vi "Utilization.vi"() -> ()   [LabVIEW 2012]
uses:
  <vilib>/addons/database/Auxilliary.llb/DB Tools Cursor Type.ctl
  <vilib>/addons/database/Connection.llb/DB Tools Open Connec (Path).vi
  <vilib>/addons/database/Connection.llb/Conn Execute.vi
  <vilib>/addons/database/Recordset.llb/Rec Fetch Recordset Data (R).vi
  <vilib>/addons/database/Recordset.llb/Rec Destroy - Connection.vi
  <vilib>/addons/database/_DB Variant To Data/Database Variant To Data.xnode
  <vilib>/addons/database/NI_Database_API.lvlib
panel:
  out "sum":dbl
  out "array":dbl[](array[numeric])
  out "data 6":string
  out "Minutes 3":i32
  out "Minutes 2":i32
  out "Numeric 2":i32
  out "Numeric":i32
  out "Minutes":i32
  out "data 5":string
  out "data 4":string
  out "data 3":string
  out "data 2":string
  out "data":string
  out "recordset data":variant[][](array[variant])
  out "error out":errorcluster
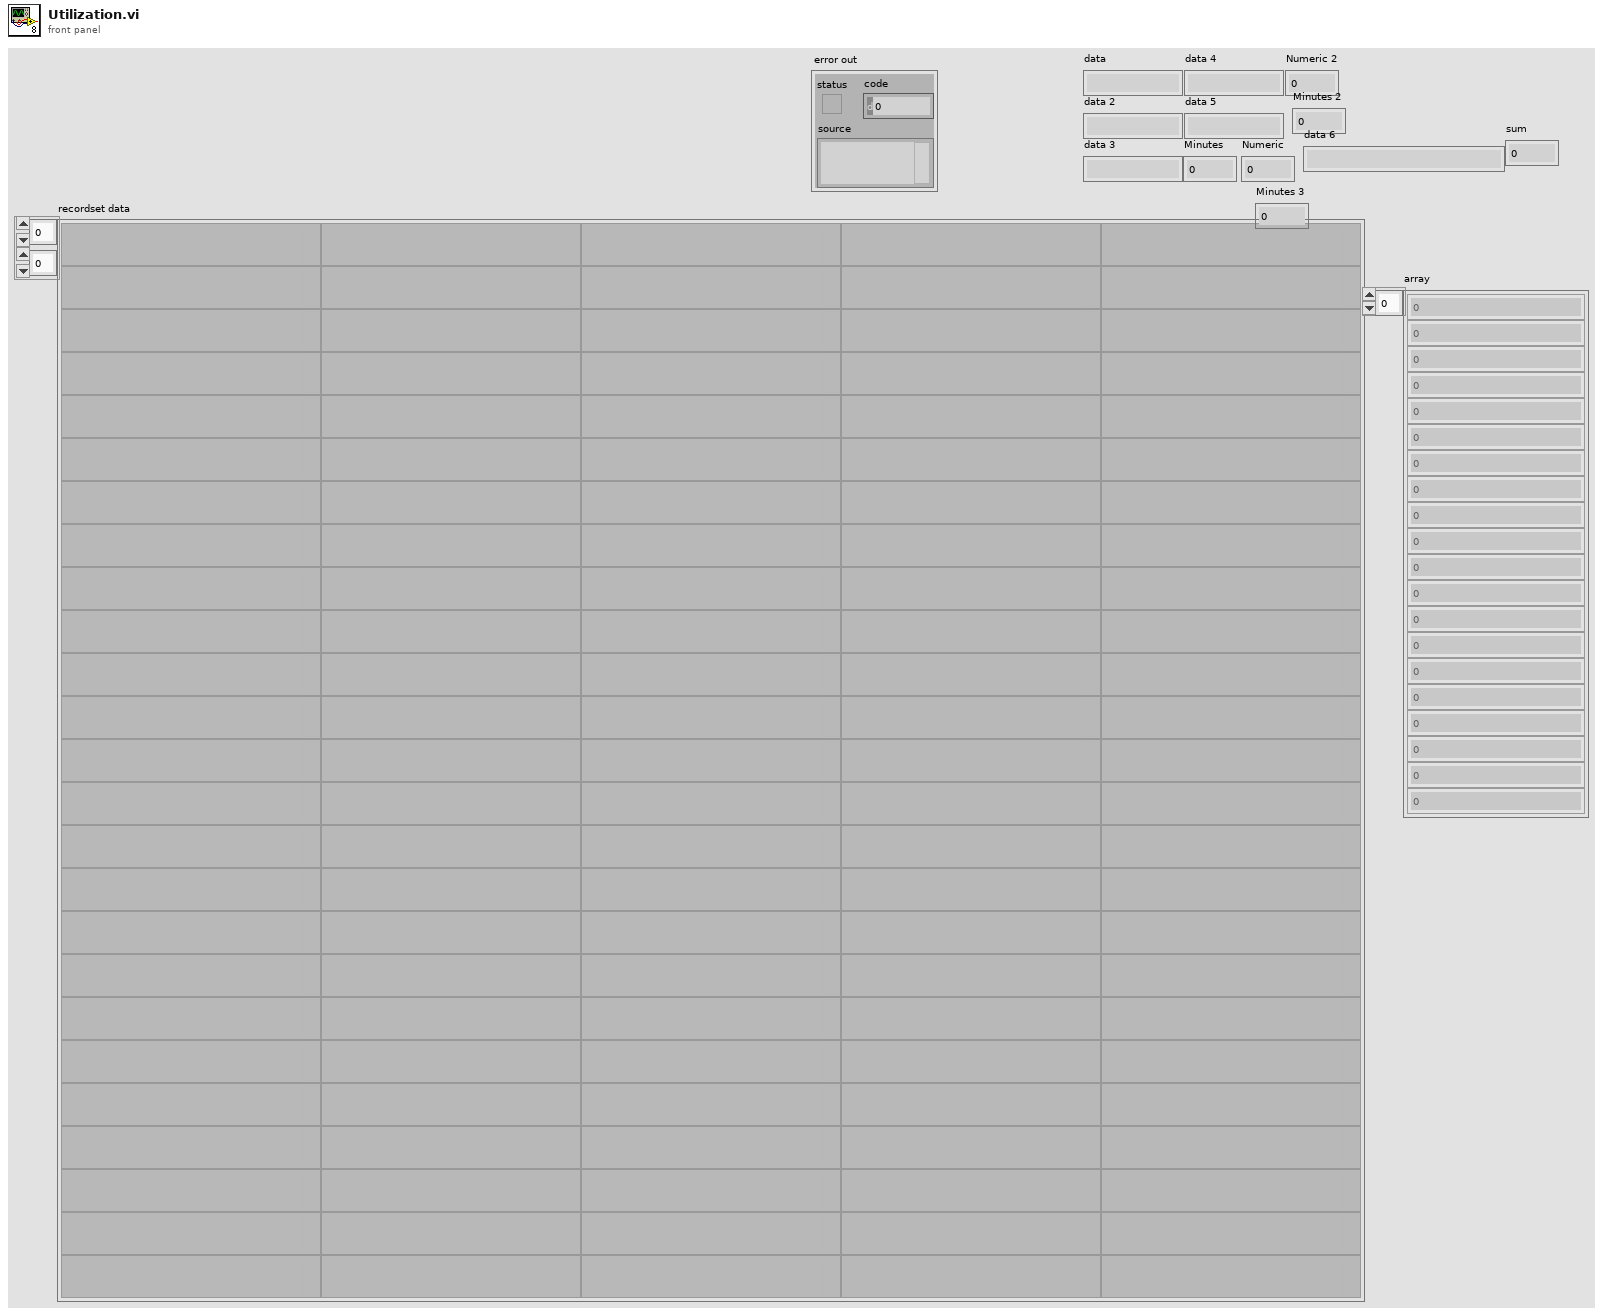
[diagram p1: front panel]
types:
  T1 = typedef "NI_Database_API.lvlib/DB Tools Cursor Type.ctl" = enum16{"forward-only", "keyset", "dynamic", "static"}
  T2 = typedef "NI_Database_API.lvlib/Conn ObjectReference.ctl" = refnum<k1>
  T3 = typedef "NI_Database_API.lvlib/Rec ObjectReference.ctl" = refnum<k1>
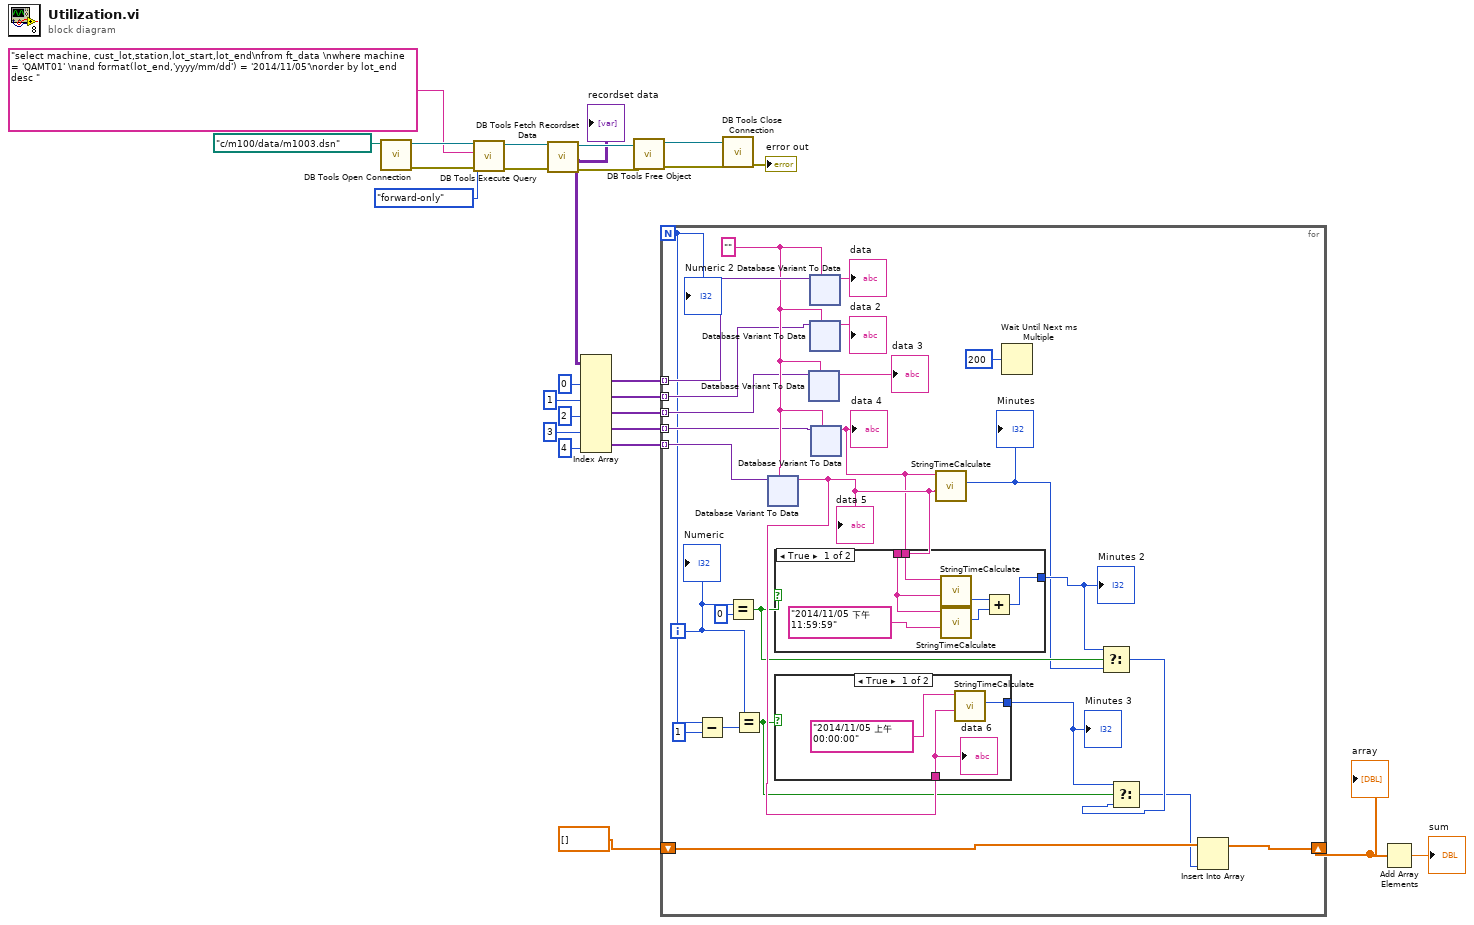
[diagram p0: block diagram]
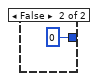
[diagram p2: hidden frame]
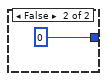
[diagram p3: hidden frame]
diagram:
  n1 = call-poly <vilib>:"DB Tools Open Connection.vi"("connection information"=path "c:/m100/data/m1003.dsn") -> ("error out"=w20:errorcluster, "connection reference"=w25:T2)  [unwired: 7 in]
  n2 = call-poly <vilib>:"DB Tools Execute Query.vi"("error in (no error)"=w20, "cursor type"=DB_Tools_Cursor_Type."forward-only", "SQL query"="select machine, cust_lot,station,lot_start,lot_end\nfrom ft_data \nwhere machine = 'QAMT01' \nand format(lot_end,'yyyy/mm/dd') = '2014/11/05'\norder by lot_end  desc ", "connection reference"=w25) -> ("error out"=w19:errorcluster, "recordset reference"=w24:T3)  [unwired: 4 in]
  n3 = call-poly <vilib>:"DB Tools Fetch Recordset Data.vi"("error in (no error)"=w19, "recordset reference"=w24) -> ("error out"=w18:errorcluster, "recordset data"=w14:variant[][], "recordset reference out"=w23:T3)  [unwired: 3 in]
  "recordset data" <- w14
  n4 = Index Array(array=w14, index (col) #1=0 ("disabled index (col)"), index (col) #2=1 ("index (col)"), index (col) #3=2 ("index (col)"), index (col) #4=3 ("index (col)"), index (col) #5=4 ("index (col)")) -> (element #1=w8:variant[], element #2=w7:variant[], element #3=w6:variant[], element #4=w5:variant[], element #5=w4:variant[])  [unwired: 5 in]
  n5 = call-poly <vilib>:"DB Tools Free Object.vi"("error in (no error)"=w18, "recordset reference"=w23) -> ("error out"=w17:errorcluster, "connection reference"=w22:T2)  [unwired: 8 in]
  n6 = for {
    N -> [w39]
    tunnel: w8 -> [w52] mode=indexing
    tunnel: w7 -> [w50] mode=indexing
    tunnel: w6 -> [w49] mode=indexing
    tunnel: w5 -> [w48] mode=indexing
    tunnel: w4 -> [w47] mode=indexing
    shift-right: [w36] -> w2
    shift-left: dbl[] [] ("array") -> [w35]
    i -> [w41]
    w51 = ""
    n7 = Subtract(x=w39, y=1) -> (x-y=w40:i32)
    n8 = Equal?(x=w41, y=0) -> (x = y?=w34:bool)
    n9 = Equal?(x=w41, y=w40) -> (x = y?=w32:bool)
    n10 = xnode "Database Variant To Data"("database variant"=w47, "type"=w51) -> ("data"=w37:string)  [unwired: 1 in, 1 out]
    "data 5" <- w37
    n11 = case shown="True" w32 {
      tunnel: [w55 0 ("Minutes")] -> w31
      tunnel: w37 -> [w53 _]
      frame True {
        n12 = call "StringTimeCalculate.vi"("End Date"=w53, "Start Date"="2014/11/05 上午 00:00:00") -> ("Minutes"=w55:i32)  [unwired: 9 in]
        "data 6" <- w53
      }
      frame False {
      }
    }
    "Minutes 3" <- w31
    n13 = xnode "Database Variant To Data"("database variant"=w49, "type"=w51) -> ("data"=→"data 3":string)  [unwired: 1 in, 1 out]
    n14 = xnode "Database Variant To Data"("database variant"=w52, "type"=w51) -> ("data"=→"data":string)  [unwired: 1 in, 1 out]
    n15 = xnode "Database Variant To Data"("database variant"=w50, "type"=w51) -> ("data"=→"data 2":string)  [unwired: 1 in, 1 out]
    n16 = xnode "Database Variant To Data"("database variant"=w48, "type"=w51) -> ("data"=w27:string)  [unwired: 1 in, 1 out]
    "data 4" <- w27
    n17 = case shown="True" w34 {
      tunnel: w37 -> [w61 _]
      tunnel: [w57 0 ("Minutes")] -> w33
      tunnel: w27 -> [w60 _]
      frame True {
        n18 = call "StringTimeCalculate.vi"("End Date"=w61, "Start Date"=w60) -> ("Minutes"=w58:i32)  [unwired: 9 in]
        n19 = call "StringTimeCalculate.vi"("End Date"="2014/11/05 下午 11:59:59", "Start Date"=w61) -> ("Minutes"=w59:i32)  [unwired: 9 in]
        n20 = Add(x=w58, y=w59) -> (x+y=w57:i32)
      }
      frame False {
      }
    }
    "Minutes 2" <- w33
    n21 = call "StringTimeCalculate.vi"("End Date"=w37, "Start Date"=w27) -> ("Minutes"=w30:i32)  [unwired: 9 in]
    "Minutes" <- w30
    n22 = Wait Until Next ms Multiple(millisecond multiple=u32 200) -> ()  [unwired: 1 out]
    n23 = Select(t=w33, s=w34, f=w30) -> (s? t:f=w29:i32)
    n24 = Select(t=w31, s=w32, f=w29) -> (s? t:f=w28:i32)
    n25 = Insert Into Array(array=w35, new element=w28) -> (w36:dbl[])  [unwired: 1 in]
    "Numeric" <- w41
    "Numeric 2" <- w39
  }
  "array" <- w2
  n26 = call <vilib>:"DB Tools Close Connection.vi"("error in (no error)"=w17, "connection reference"=w22) -> ("error out"=→"error out":errorcluster)  [unwired: 5 in]
  n27 = Add Array Elements(numeric array=w2) -> (sum=→"sum":dbl)
